vi "FID Main.vi"(8 "error in (no error)":errorcluster, 11 "User information":T1) -> (0 "error out":errorcluster)   [LabVIEW 2020]
uses:
  Controls/1775E_Authen_Level.ctl
  Controls/user_log.ctl
  <vilib>/Utility/miscctls.llb/LVPointTypeDef.ctl
  Controls/User_DB.ctl
  <vilib>/Instr/_visa.llb/VISA Configure Serial Port (Instr).vi
  <vilib>/addons/database/Connection.llb/Conn Execute.vi
  <vilib>/addons/database/Recordset.llb/Rec Fetch Recordset Data (R).vi
  <vilib>/addons/database/Recordset.llb/Rec Destroy - Connection.vi
  <vilib>/addons/database/NI_Database_API.lvlib
panel:
  in  "Hide":bool
  in  "Auth. Password":string caption="Password"
  in  "Change Password":bool
  out "State":string
  out "Device Info":string
  out "Numeric":i32
  in  "Re-enter Password":string
  in  "Password":string caption="New Password"
  in  "View Log":bool
  out "Cmd.":bool
  in  "Super User":bool
  in  "View All":bool
  out "String":string
  out "data":T1
  in  "Clock No.":string
  in  "Level":T2
  in  "User Name":string
  in  "ID Number":i16
  out "Finger Present?":bool
  out "Response":string
  in  "Delete All":bool
  in  "Delete":bool
  in  "Search":bool
  in  "Enroll":bool
  out "Status":string
  out "elements":u8[](array[numeric]) format="%.0x"
  in  "Stop":bool
  out "Buffer Out":string
  in  "write buffer":string="ï\u0001ÿÿÿÿ\u0001\u0000\u00034\u00008"
  out "Profile Image":picture
  in  "Image Location":path
  # "User Access Control"
  # "thumb finger"
  # "EF01 FFFF FFFF 0700 0700 0003 00A4 00B5"
  # "EF01 FFFF FFFF 0700 0709 0003 0028 0042"
  # "EF01 FFFF FFFF 0700 0700 0000 0065 0073"
  # "EF01 FFFF FFFF 0700 0700 0001 0084 0093"
  # "EF01 FFFF FFFF 0700 0709 0003 0002 001C"
  # "wrong finger"
  # "EF01 FFFF FFFF 0700 0703 0000 0000 0011"
  # "NO finger"
  # "EF01 FFFF FFFF 0700 0703 0000 0000 0011"
  # "EF01 FFFF FFFF 0700 0703 0000 0000 0011"
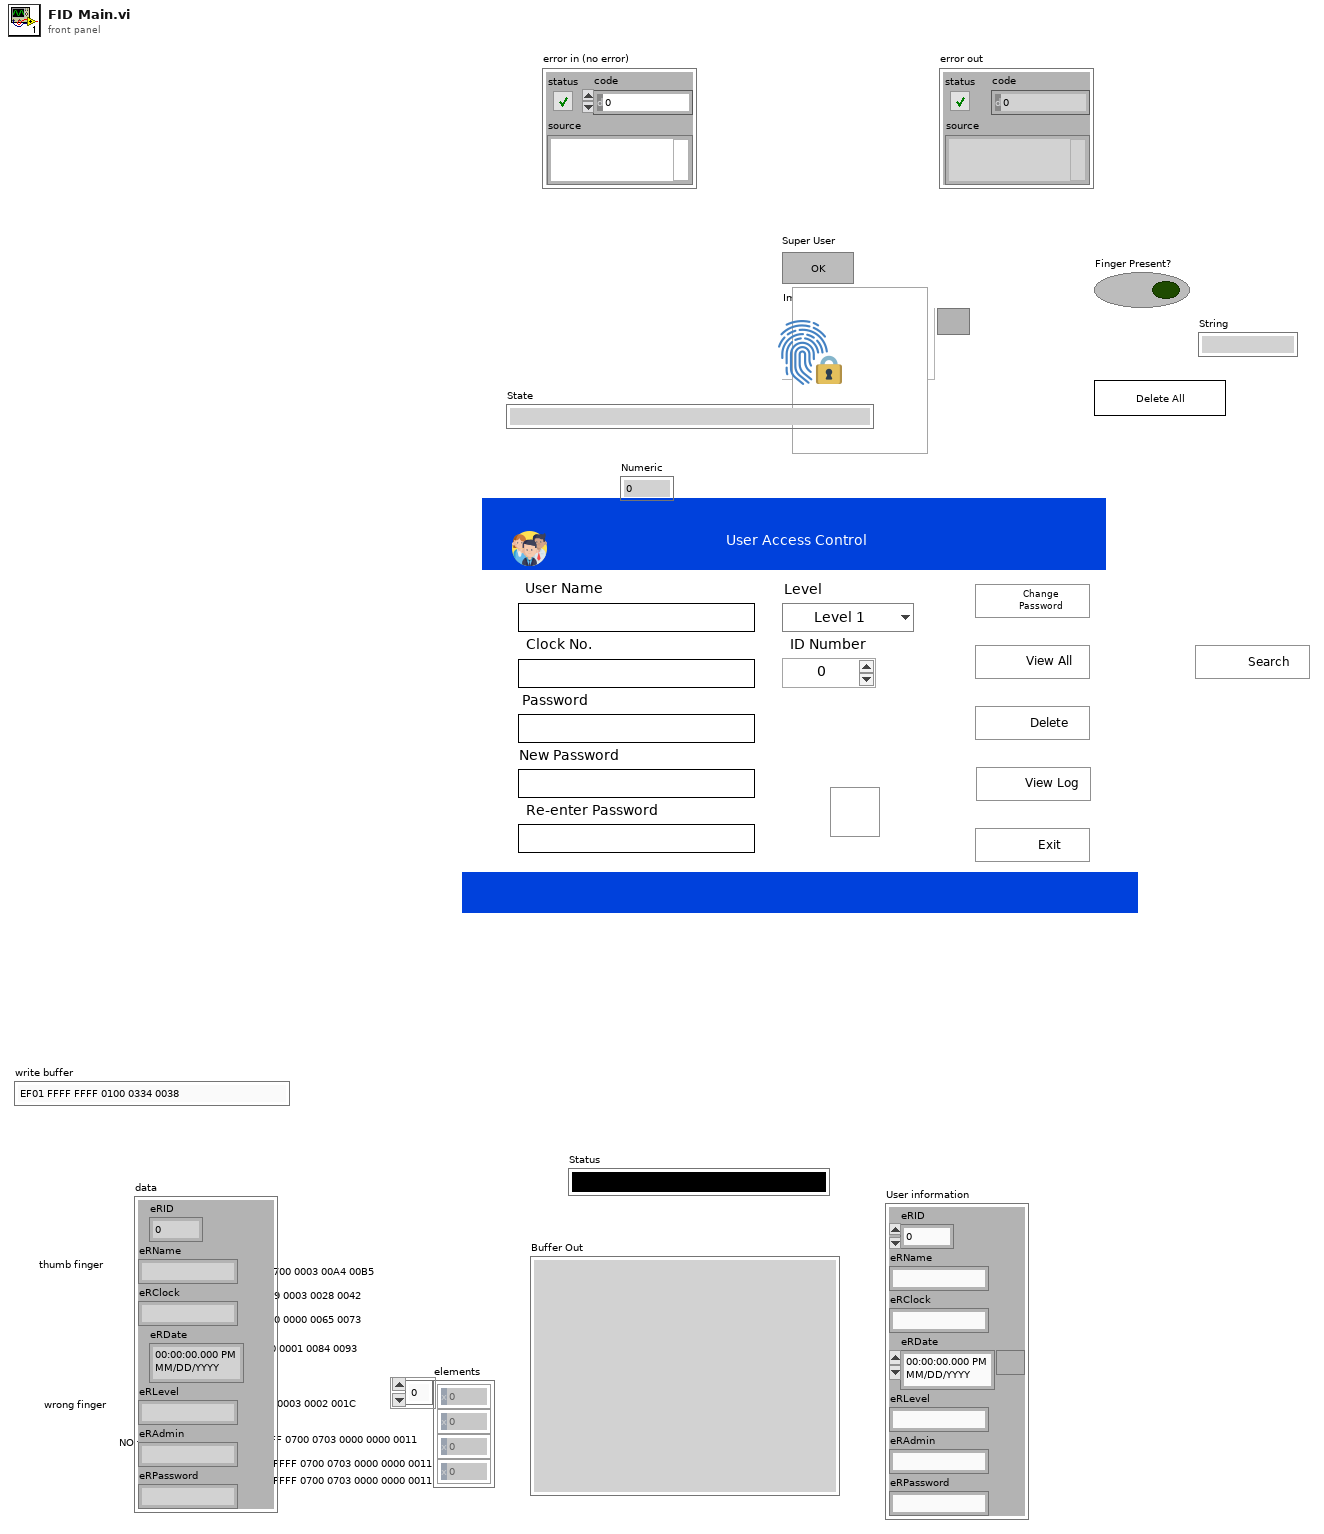
[diagram p1: front panel]
types:
  T1 = typedef "user_log.ctl" = cluster{"eRID":u16, "eRName":string, "eRClock":string, "eRDate":timestamp, "eRLevel":string, "eRAdmin":string, "eRPassword":string}
  T2 = typedef "1775E_Authen_Level.ctl" = enum16{"Level 1", "Level 2", "Level 3", "Level 4", "Super Level"}
  T3 = typedef "LVPointTypeDef.ctl" = cluster{"Horizontal":i16, "Vertical":i16}
  T4 = typedef "TD SQL.ctl" = cluster{"MS SQL Connection":T5, "UDL File":path, "Time":string, "DCODE":string, "WIP+1":i64, "MC No?":i32, "POKAYOKE?":bool, "Expected Result":string, "Result [Status]":string, "Clock":dbl, "RFID":string, "WIP Queue":refnum<queue>, "TS Parameter":T6, "Data_Queue":refnum<queue>[], "RFID Serial No.":string}
  T5 = typedef "NI_Database_API.lvlib/Conn ObjectReference.ctl" = refnum<k1>
  T6 = typedef "TS_Parameter.ctl" = cluster{"ProfitCenterCode":string, "LineCode":string, "WorkOrderNumber":string, "Model":string, "Model_with_Prefix":string, "VendorCode":string, "SetParameterDateCode":string, "PokaYoke":i32, "Target":i32, "Live_DateCode":string, "CustomerPartNumber":string, "Hand":string, "sBarcode":bool, "FCA":i32, "Ent_Stamp":timestamp, "STS_CD":dbl}
  T7 = typedef "User_DB.ctl" = cluster{"eRID":u16, "eRName":string, "eRClock":string, "eRDate":timestamp, "eRLevel":string, "eRAdmin":string, "eRPassword":string, "eRPurpose":string}
  T8 = typedef "NI_Database_API.lvlib/Rec ObjectReference.ctl" = refnum<k1>
  T9 = typedef "imagedata.ctl" = cluster{"image type":i32, "image depth":i32, "image":u8[], "mask":u8[], "colors":u32[], "Rectangle":cluster{"left":i16, "top":i16, "right":i16, "bottom":i16}}
  T10 = typedef "LVBoundsTypeDef.ctl" = cluster{"Width":u32, "Height":u32}
  T11 = cluster{"left":i16, "top":i16, "right":i16, "bottom":i16}
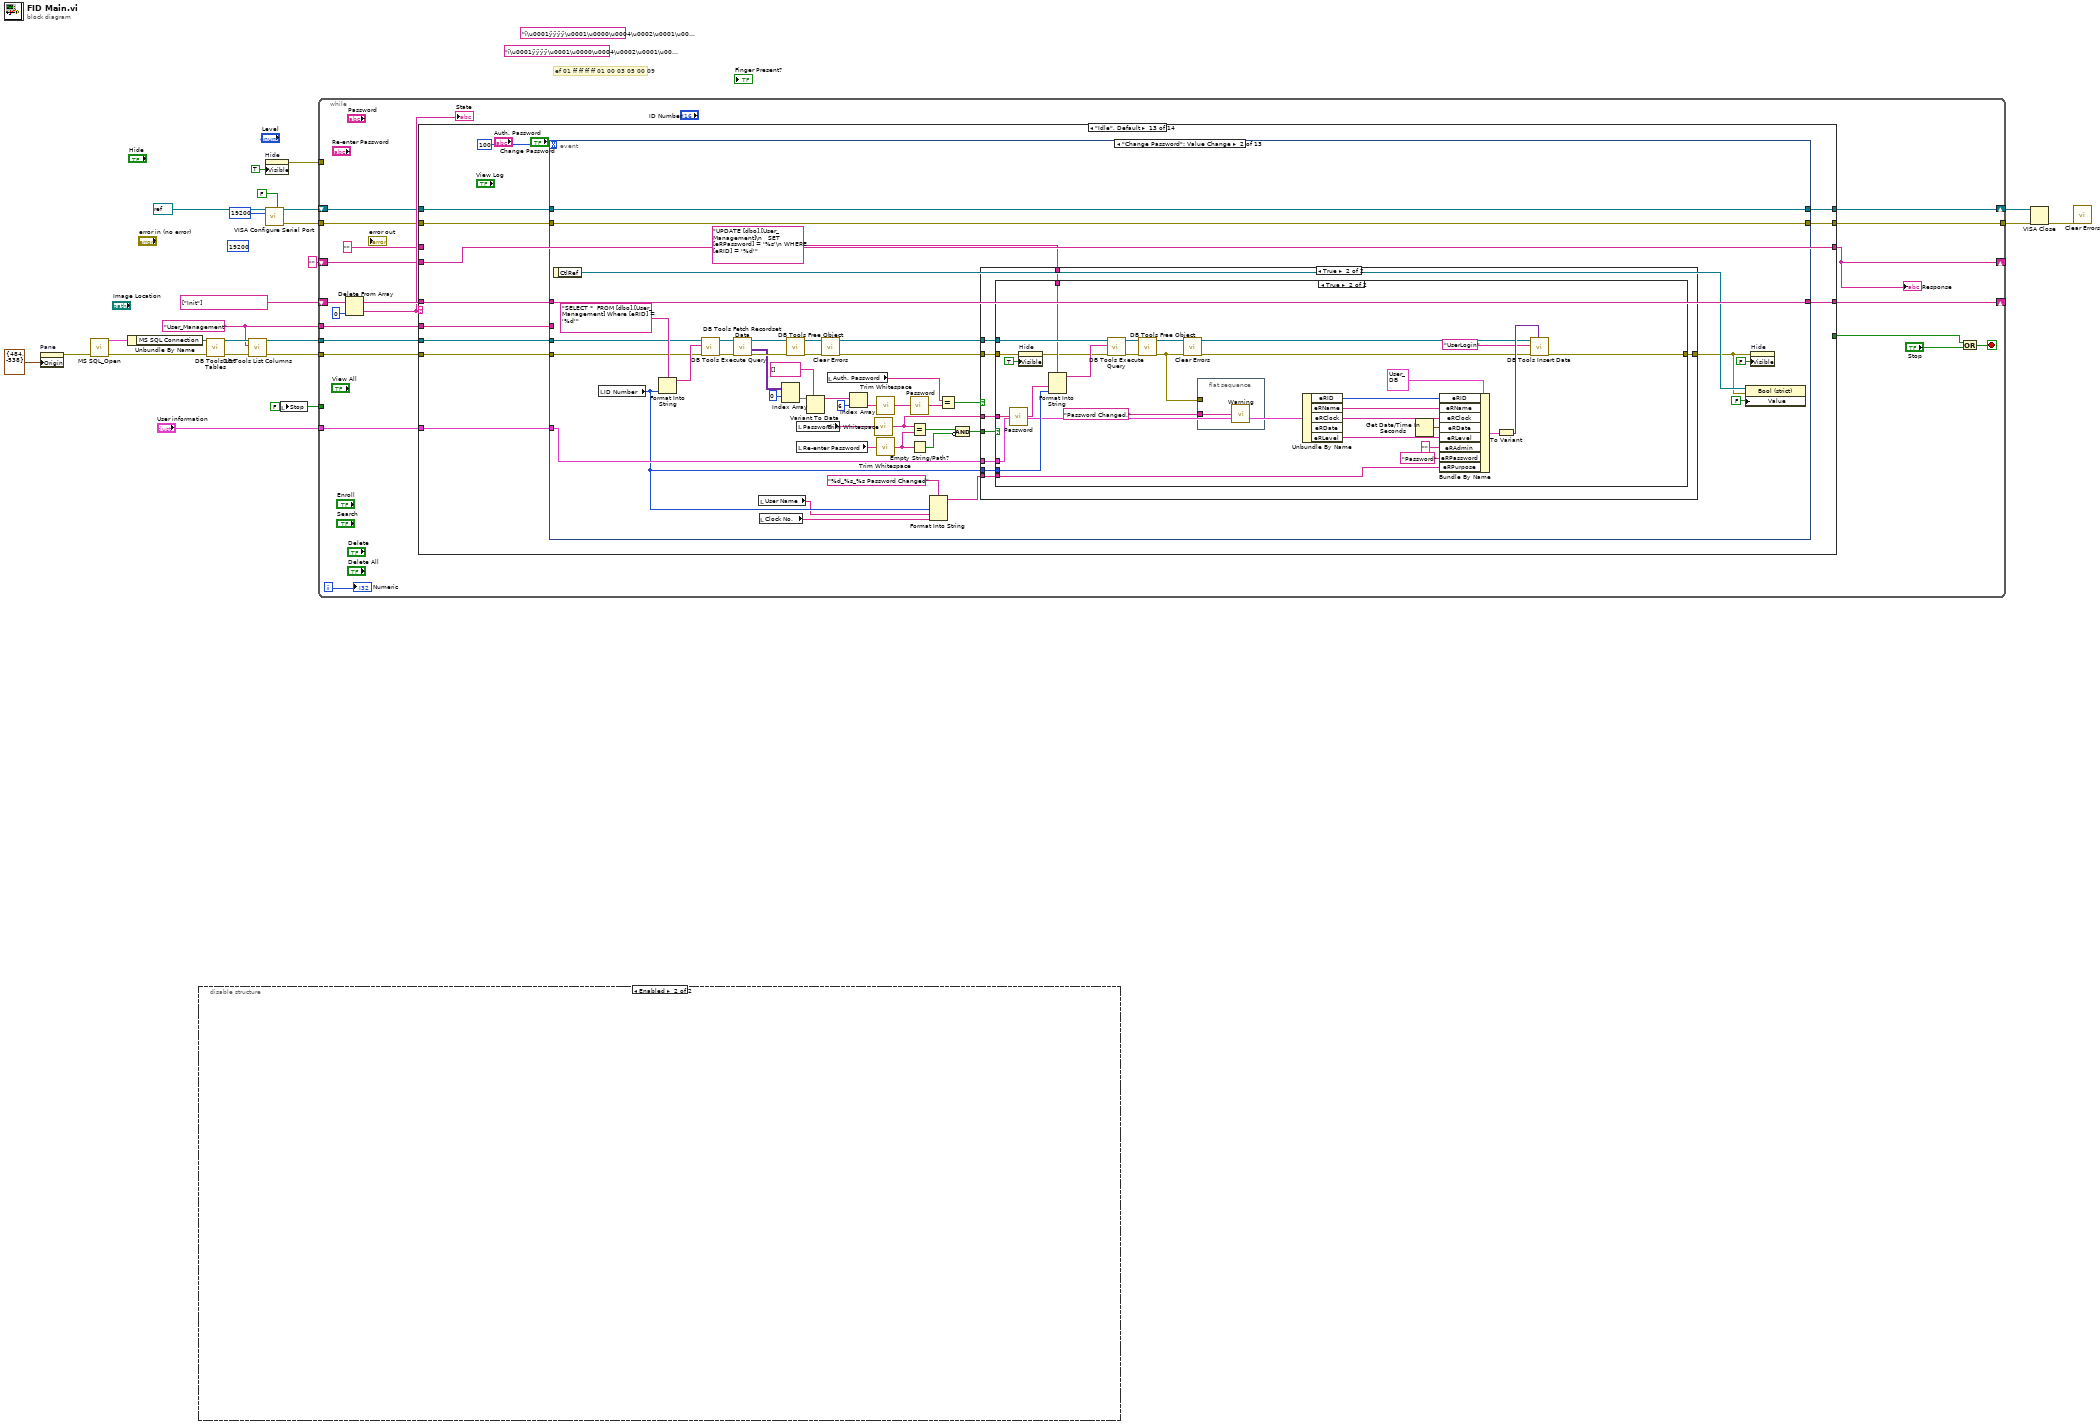
[diagram p0: block diagram]
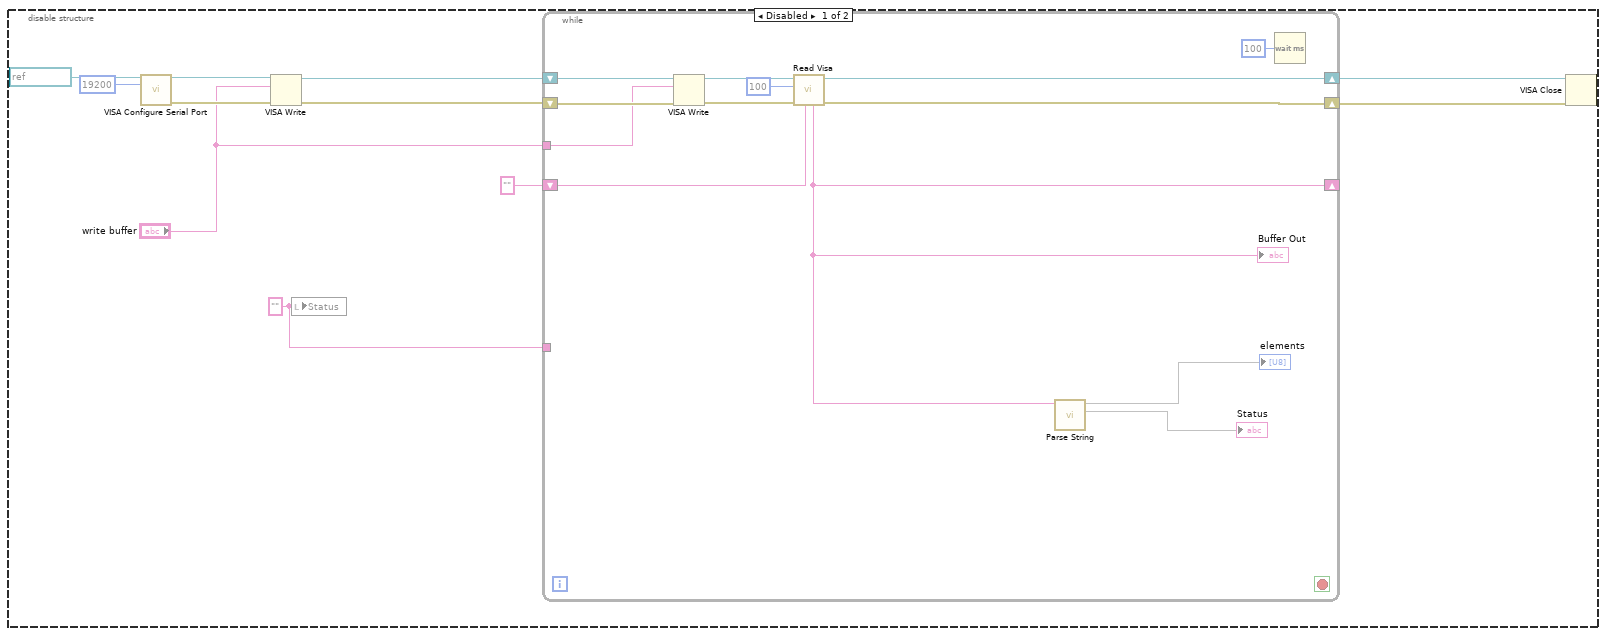
[diagram p2: hidden frame]
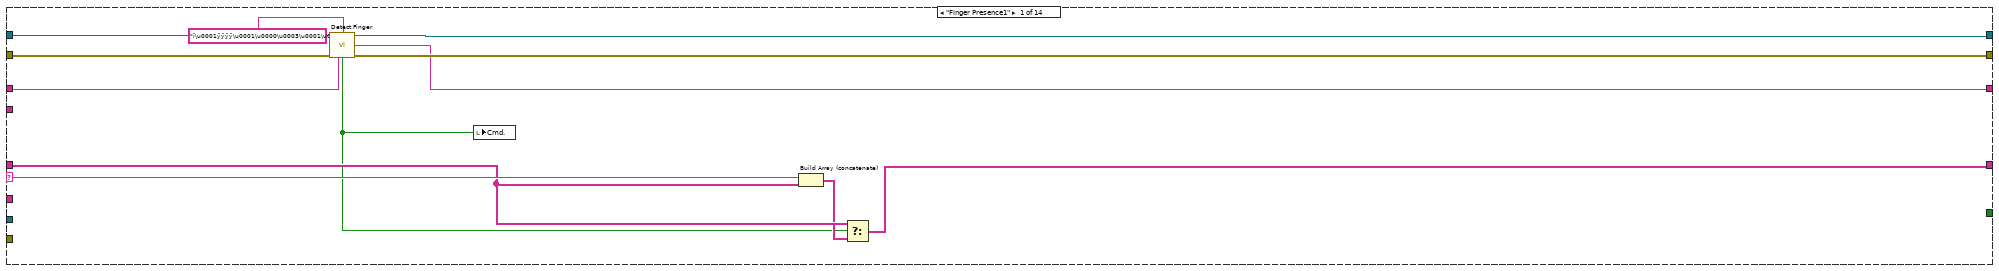
[diagram p3: hidden frame]
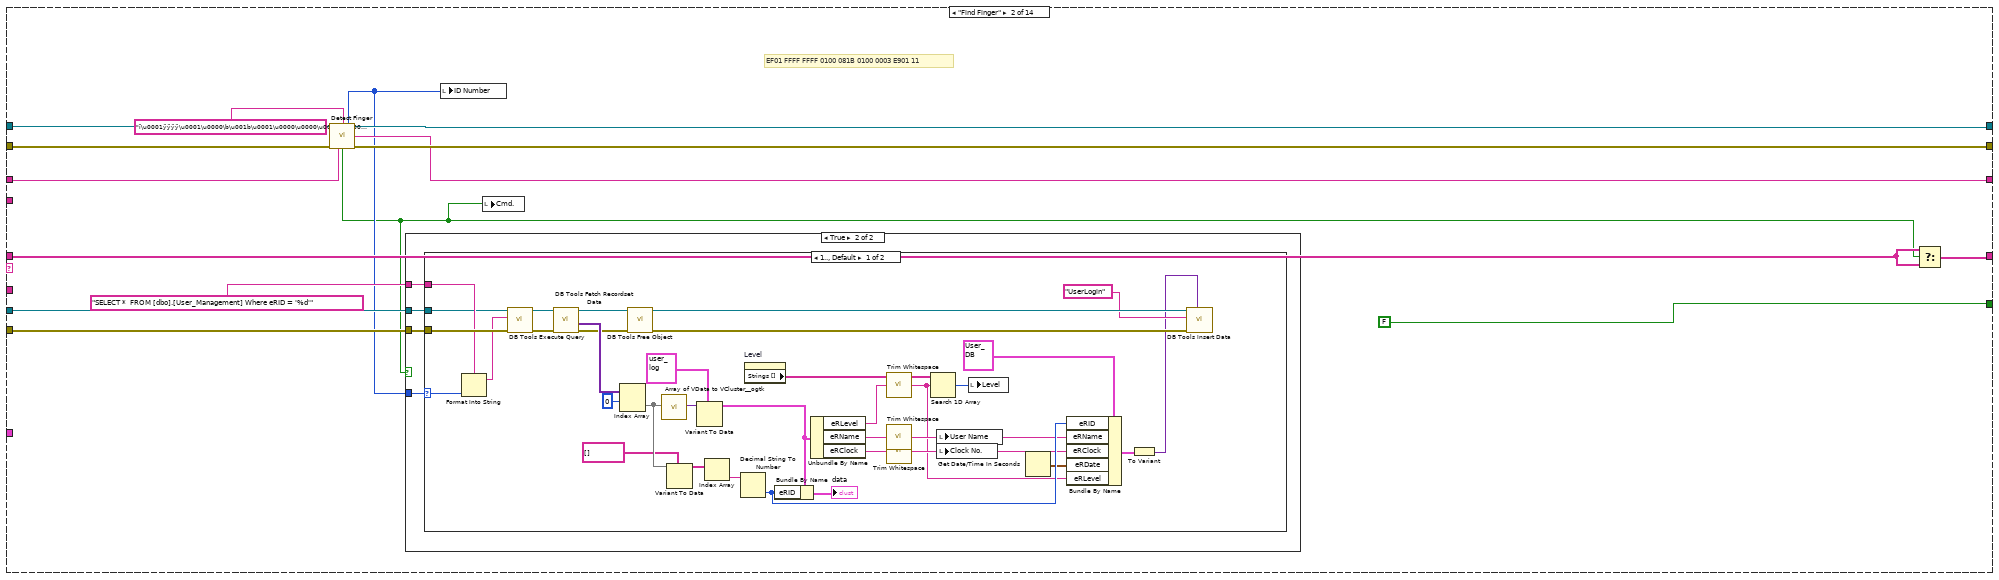
[diagram p4: hidden frame]
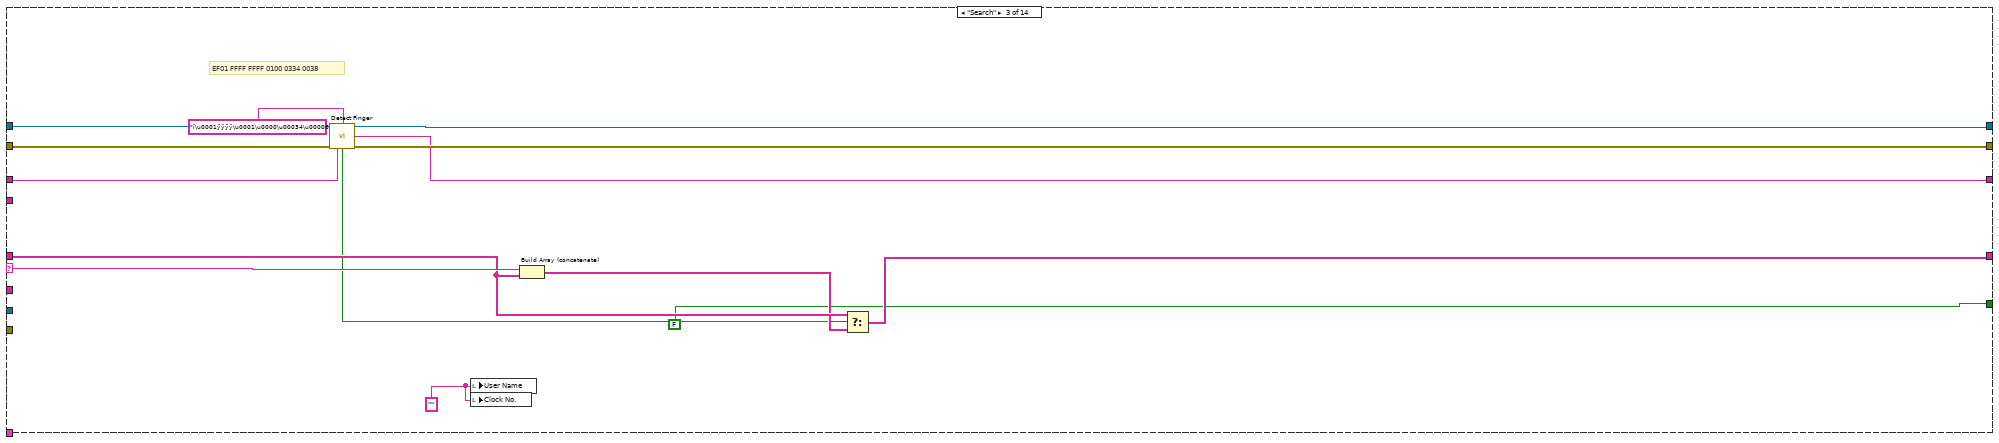
[diagram p7: hidden frame]
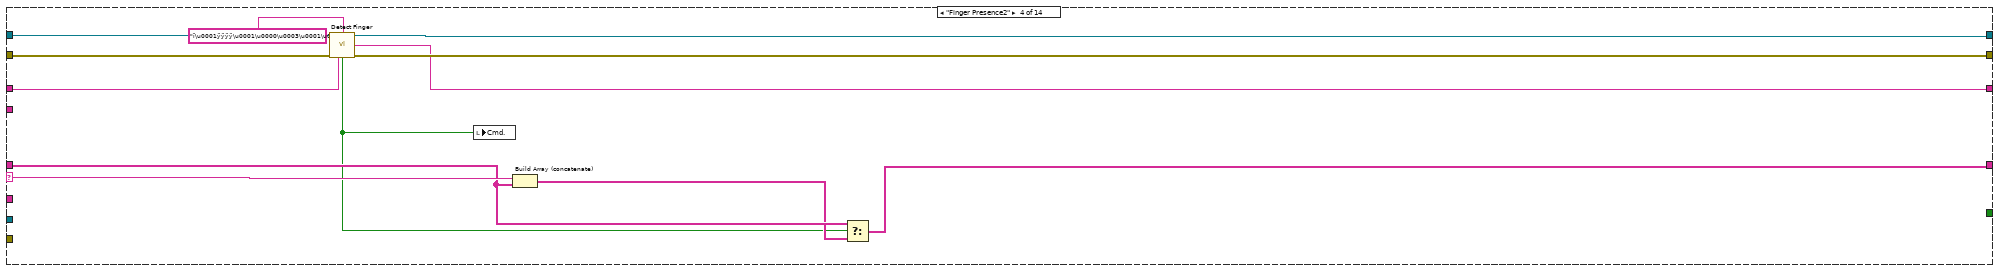
[diagram p8: hidden frame]
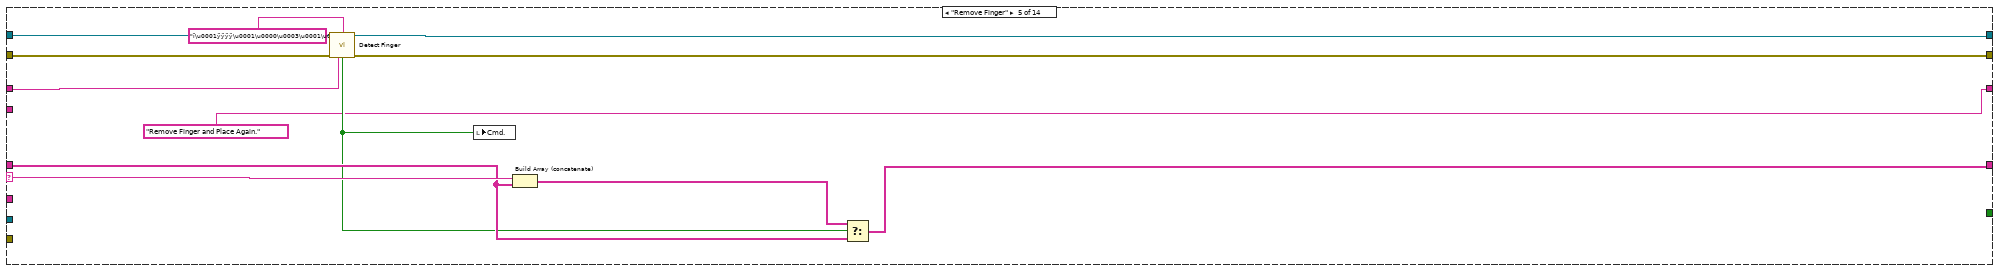
[diagram p9: hidden frame]
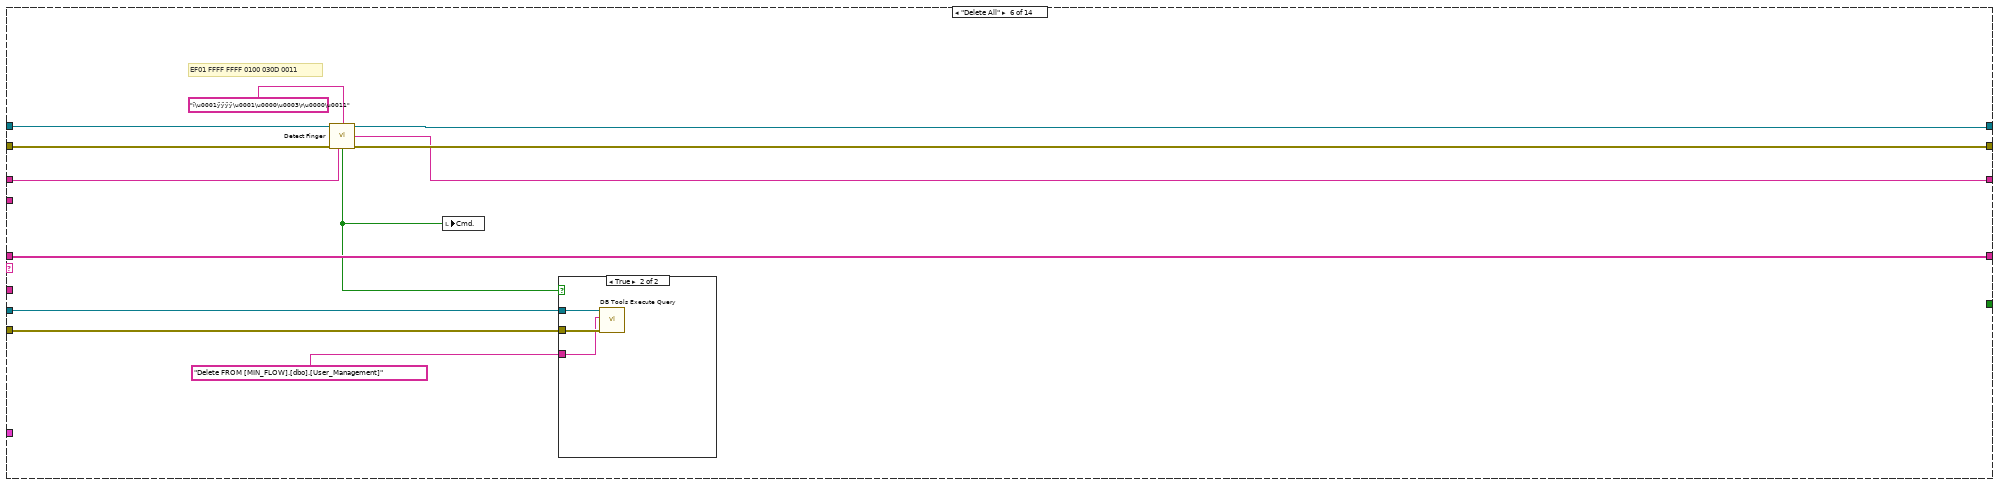
[diagram p10: hidden frame]
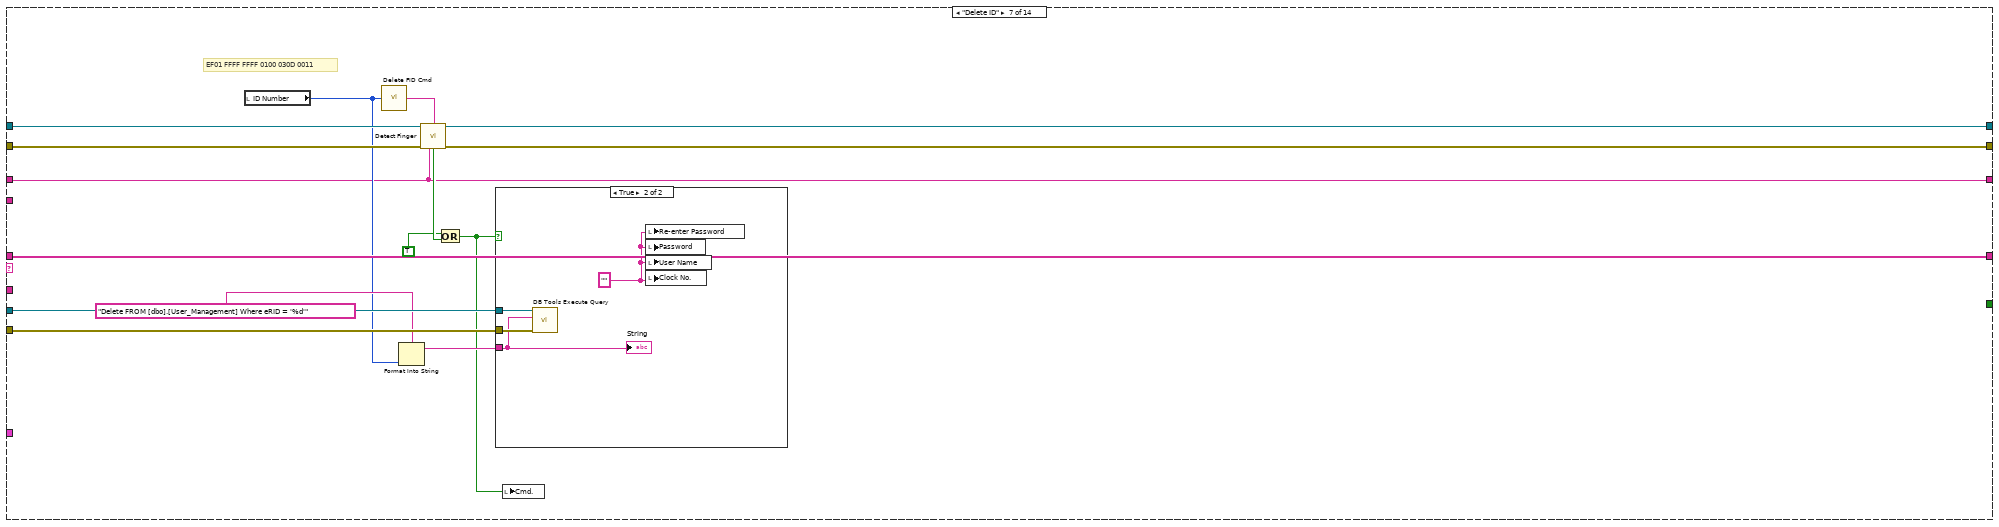
[diagram p12: hidden frame]
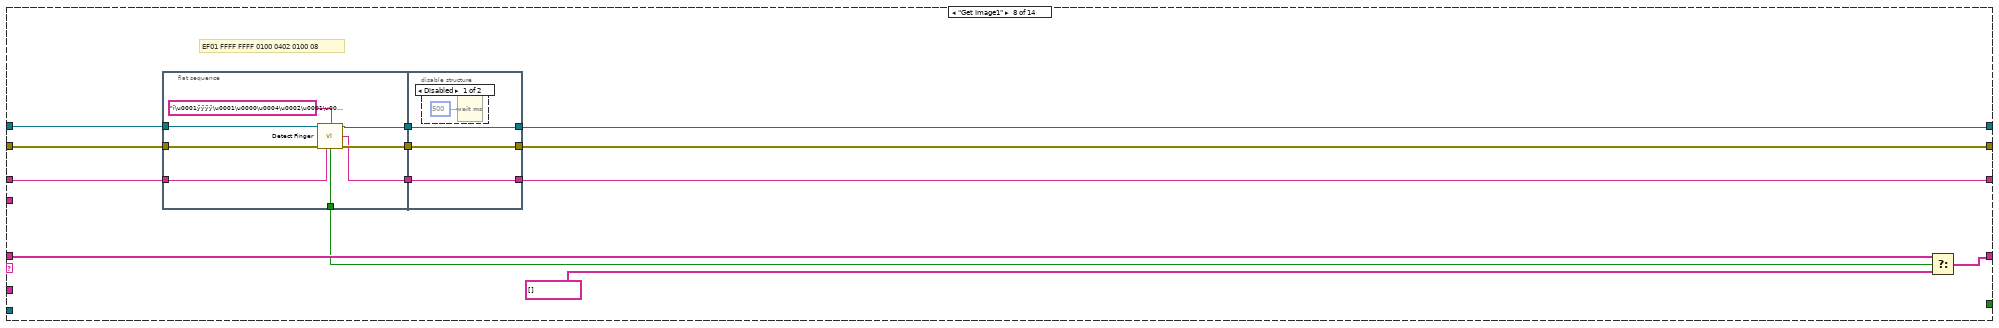
[diagram p14: hidden frame]
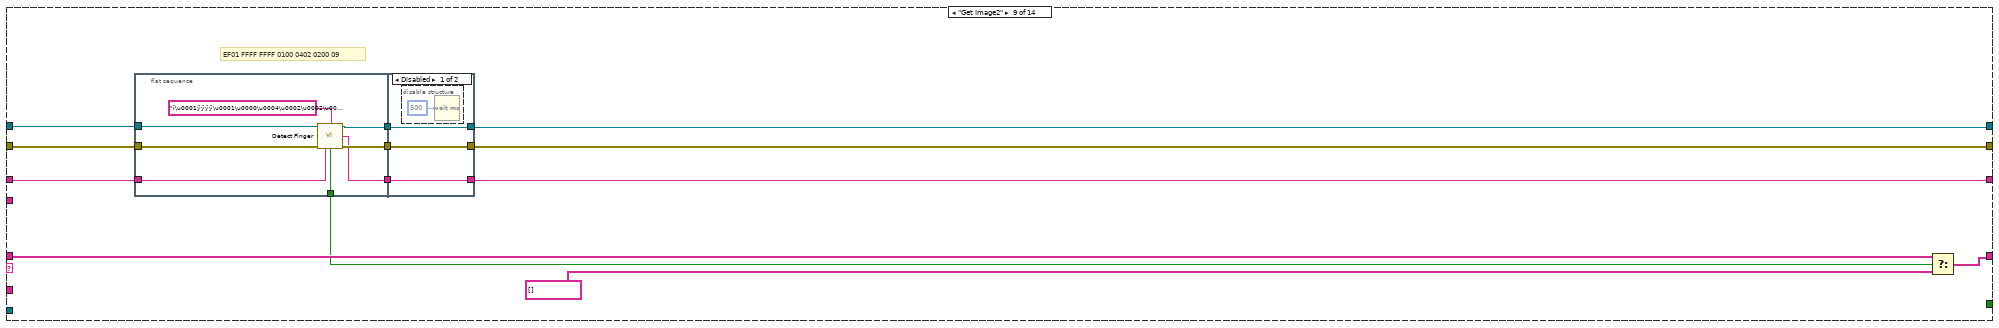
[diagram p16: hidden frame]
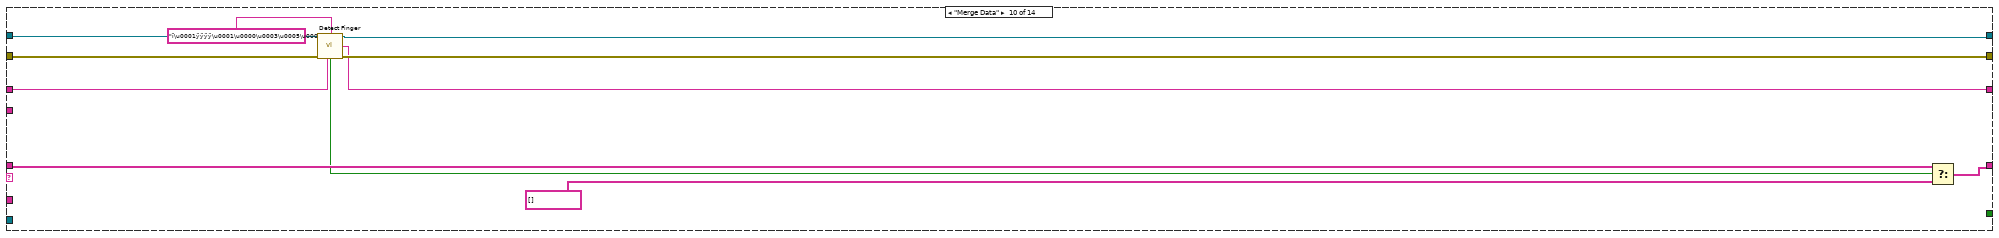
[diagram p18: hidden frame]
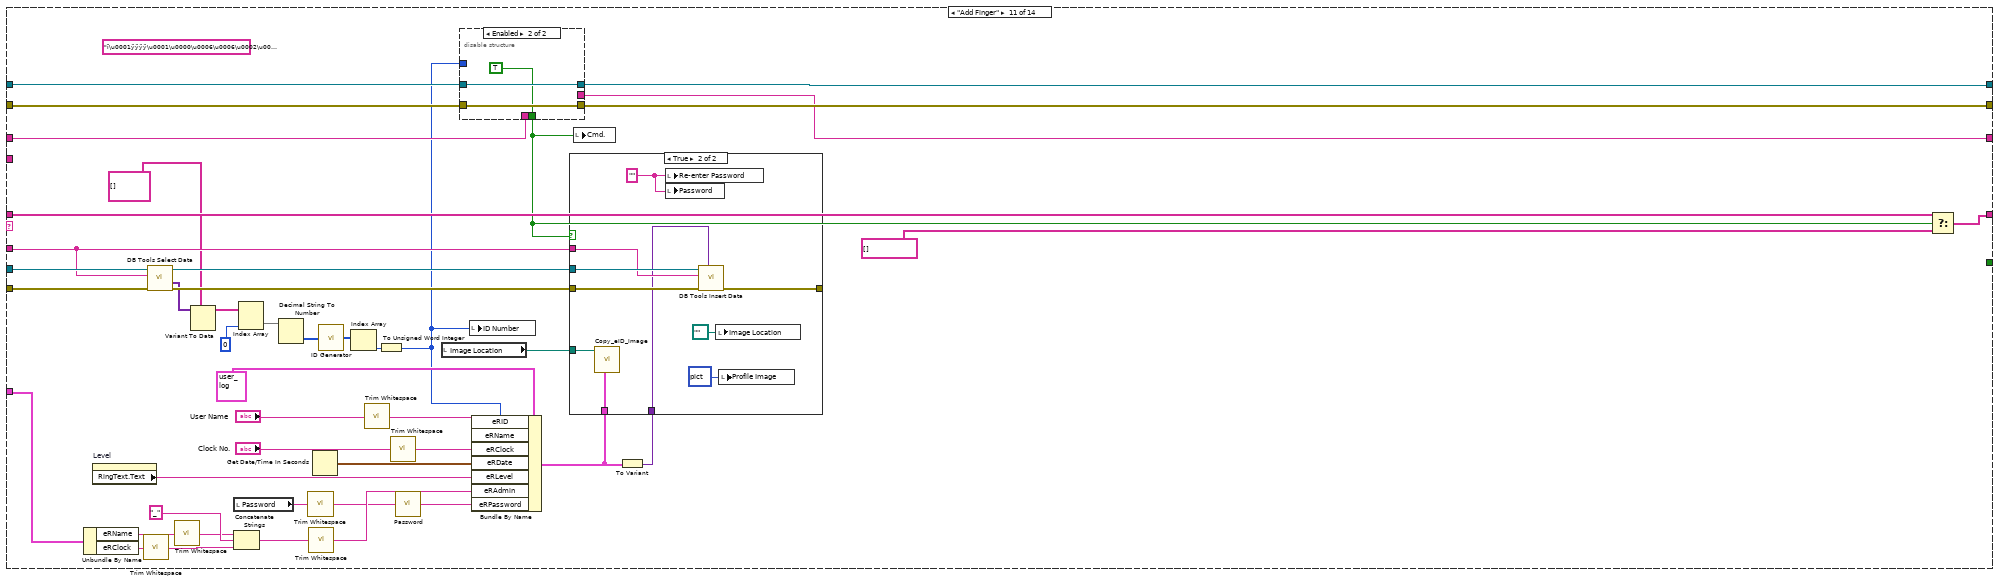
[diagram p19: hidden frame]
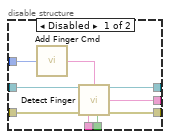
[diagram p20: hidden frame]
diagram:
  (unwired) u32 19200 ("baud rate (9600)")
  w11 = FALSE ("Stop")
  w12 = "User_Management" ("table")
  (unwired) "ï\u0001ÿÿÿÿ\u0001\u0000\u0004\u0002\u0001\u0000\b" ("write buffer")
  (unwired) "ï\u0001ÿÿÿÿ\u0001\u0000\u0004\u0002\u0001\u0000\b" ("write buffer")
  # "ef 01 ff ff ff ff 01 00 03 05 00 09"
  n1 = property on="Pane" class="Pane"("Origin"=T3 {"Horizontal"=484, "Vertical"=-538}) -> (error out=w2:errorcluster)  [unwired: 2 in, 1 out]
  n2 = call "MS SQL_Open.vi"("error in (no error)"=w2) -> ("error out"=w1:errorcluster, "Ref Out"=w4:T4)  [unwired: 8 in, 1 out]
  n3 = Unbundle By Name(w4) -> ("MS SQL Connection"=w3:T5)
  n4 = disable-structure shown="Enabled" {
    frame Disabled {
      w25 = "" ("Status")
      n5 = call-poly "VISA Configure Serial Port"("VISA resource name"=refnum<visa-resource-name> "COM6", "baud rate (9600)"=u32 19200) -> ("VISA resource name out"=w31:refnum<visa-resource-name>, "error out"=w29:errorcluster)  [unwired: 12 in]
      n6 = VISA Write(VISA resource name=w31, write buffer="write buffer", error in (no error)=w29) -> (VISA resource name out=w30:refnum<visa-resource-name>, error out=w28:errorcluster)  [unwired: 1 out]
      n7 = local write "Status"(w25) -> ()
      n8 = while {
        shift-right: [w49] -> w33
        shift-left: w30 -> [w43]
        shift-right: [w48] -> w32
        shift-left: w28 -> [w42]
        shift-right: [w38] -> _
        shift-left: "" ("Buffer Out") -> [w44]
        tunnel: "write buffer" -> [w39]
        tunnel: w25 -> [_]
        stop <- w46 stop-if-true
        n9 = VISA Write(VISA resource name=w43, write buffer=w39, error in (no error)=w42) -> (VISA resource name out=w40:refnum<visa-resource-name>, error out=w41:errorcluster)  [unwired: 1 out]
        n10 = call <userlib>:"Read Visa.vi"("Buffer In"=w44, "error in (no error)"=w41, "delay before read (ms)"=u32 100, "VISA Refnum in"=w40) -> ("error out"=w48:errorcluster, "VISA Refnum out"=w49:refnum<visa-resource-name>, "Buffer Out"=w38:string)  [unwired: 5 in]
        "Buffer Out" <- w38
        n11 = call "Parse String.vi"("Ack package"=w38) -> (2:→"Status", 3:→"elements")  [unwired: 7 in, 2 out]
        n12 = Wait (ms)(milliseconds to wait=u32 100) -> ()  [unwired: 1 out]
      }
      n13 = VISA Close(VISA resource name=w33, error in (no error)=w32) -> ()  [unwired: 1 out]
    }
    frame Enabled {
    }
  }
  n14 = call <vilib>:"DB Tools List Tables.vi"("error in (no error)"=w1, "connection reference"=w3) -> ("error out"=w15:errorcluster, "connection reference out"=w16:T5)  [unwired: 3 in, 1 out]
  n15 = call <vilib>:"DB Tools List Columns.vi"("error in (no error)"=w15, "table"=w12, "connection reference"=w16) -> ("error out"=w13:errorcluster, "connection reference out"=w14:T5)  [unwired: 1 in, 2 out]
  n16 = property on="Hide" class="Bool"("Visible"=TRUE) -> (error out=w7:errorcluster)  [unwired: 2 in, 1 out]
  n17 = call-poly "VISA Configure Serial Port"("VISA resource name"=refnum<visa-resource-name> refnum, "Enable Termination\nChar (T)"=FALSE ("Enable Termination\nChar (T)"), "baud rate (9600)"=u32 19200) -> ("VISA resource name out"=w22:refnum<visa-resource-name>, "error out"=w21:errorcluster)  [unwired: 11 in]
  n18 = local write "Stop"(w11) -> ()
  n19 = while {
    shift-right: [w68] -> _
    shift-left: string[] ["Init"] -> [w69]
    tunnel: w21 -> [w51]
    shift-right: [w67] -> w19
    shift-left: w22 -> [w50]
    shift-right: [w57] -> _
    shift-left: "" ("Buffer Out") -> [w58]
    tunnel: [w64] -> w18
    tunnel: w14 -> [w56]
    tunnel: w13 -> [w55]
    tunnel: w12 -> [w54]
    tunnel: w11 -> [_]
    tunnel: "User information" -> [w53]
    tunnel: w7 -> [_]
    i -> [w52]
    stop <- w62 stop-if-true
    n20 = Delete From Array(array=w69, index=0) -> (deleted portion=w61:string, array with subset deleted=w65:string[])  [unwired: 1 in]
    "State" <- w61
    n21 = case shown="\"Idle\", Default" w61 {
      selector: w61 -> [w81 _ w149 w161 w173 _ _ _ _ _ _ _ _ _]
      tunnel: w65 -> [w80 w87 w148 w160 w172 w178 w198 w220 w245 w268 w313 w336 w350 w590]
      tunnel: [w78 w96 w146 w158 w170 w178 w198 w219 w244 w267 w312 w336 w349 w590] -> w68
      tunnel: w50 -> [w77 w95 w145 w157 w169 w185 w203 w217 w242 w265 w310 w339 w348 w588]
      tunnel: w51 -> [w76 w94 w144 w156 w168 w184 w202 w216 w241 w264 w309 w338 w347 w585]
      tunnel: [w74 w92 w142 w154 w166 w182 w200 w215 w240 w263 w308 w339 w346 w587] -> w67
      tunnel: [w75 w93 w143 w155 w167 w183 w201 w214 w239 w262 w307 w338 w345 w584] -> w64
      tunnel: [w73 w91 w141 w153 "Remove Finger and Place Again." ("Response") w181 w189 w212 w237 w260 w306 w337 w344 w589] -> w57
      tunnel: "" ("Buffer Out") -> [w70 w89 w137 w150 w163 w179 w189 w208 w233 w258 w305 w337 _ w586]
      tunnel: [_ FALSE ("Stop") FALSE ("Stop") _ _ _ _ _ _ _ _ _ _ _] -> w60
      tunnel: w58 -> [_ _ _ _ _ _ _ _ _ _ _ _ w344 _]
      tunnel: w56 -> [_ w86 _ _ _ w177 w197 _ _ _ w304 _ w343 _]
      tunnel: w55 -> [_ w85 _ _ _ w176 w196 _ _ _ w303 _ w342 _]
      tunnel: w54 -> [_ _ _ _ _ _ _ _ _ _ w299 _ w341 _]
      tunnel: w53 -> [_ _ _ _ _ _ _ _ _ _ w282 _ w340 _]
      frame "Finger Presence1" {
        n22 = call "Detect Finger.vi"("VISA Refnum in"=w77, "Cmd"="ï\u0001ÿÿÿÿ\u0001\u0000\u0003\u0001\u0000\u0005" ("write buffer"), "error in (no error)"=w76, "Buffer In"=w70) -> ("VISA Refnum out"=w74:refnum<visa-resource-name>, "Response"=w73:string, "Cmd Suceed?"=w71:bool, "error out"=w75:errorcluster)  [unwired: 6 in, 2 out]
        n23 = local write "Cmd."(w71) -> ()
        n24 = Build Array (concatenate)(w81, w80) -> (w79:string[])
        n25 = Select(t=w80, s=w71, f=w79) -> (s? t:f=w78:string[])
      }
      frame "Find Finger" {
        # "EF01 FFFF FFFF 0100 081B 0100 0003 E901 11"
        n26 = call "Detect Finger.vi"("VISA Refnum in"=w95, "Cmd"="ï\u0001ÿÿÿÿ\u0001\u0000\b\u001b\u0001\u0000\u0000\u0003é\u0001\u0011" ("write buffer"), "error in (no error)"=w94, "Buffer In"=w89) -> ("ID"=w83:i16, "VISA Refnum out"=w92:refnum<visa-resource-name>, "Response"=w91:string, "Cmd Suceed?"=w82:bool, "error out"=w93:errorcluster)  [unwired: 6 in, 1 out]
        n27 = case shown="True" w82 {
          tunnel: w86 -> [_ w100]
          tunnel: w85 -> [_ w99]
          tunnel: "SELECT *  FROM [dbo].[User_Management] Where eRID = '%d'" ("SQL query") -> [_ w98]
          tunnel: w83 -> [_ w97]
          frame False {
          }
          frame True {
            n28 = case shown="1.., Default" w97 {
              selector: w97 -> [w132 _]
              tunnel: w100 -> [w114 _]
              tunnel: w99 -> [w134 _]
              tunnel: w98 -> [w133 _]
              frame 1.., Default {
                n29 = Format Into String(format string=w133, w132) -> (resulting string=w131:string)  [unwired: 2 in, 1 out]
                n30 = call-poly <vilib>:"DB Tools Execute Query.vi"("error in (no error)"=w134, "SQL query"=w131, "connection reference"=w114) -> ("error out"=w135:errorcluster, "recordset reference"=w115:T8)  [unwired: 5 in]
                n31 = call-poly <vilib>:"DB Tools Fetch Recordset Data.vi"("error in (no error)"=w135, "recordset reference"=w115) -> ("error out"=w111:errorcluster, "recordset data"=w127:variant[][], "recordset reference out"=w113:T8)  [unwired: 3 in]
                n32 = Index Array(array=w127, index (row)=0 ("disabled index (col)")) -> (element=w126:variant[])  [unwired: 1 in]
                n33 = call-poly <vilib>:"DB Tools Free Object.vi"("error in (no error)"=w111, "recordset reference"=w113) -> ("error out"=w110:errorcluster, "connection reference"=w112:T5)  [unwired: 8 in]
                n34 = call <userlib>:"Array of VData to VCluster__ogtk.vi"("Array"=w126) -> ("VCluster"=w129:variant)  [unwired: 9 in, 1 out]
                n35 = Variant To Data(type=string[] [], Variant=w126) -> (data=w124:string[])  [unwired: 1 in, 1 out]
                n36 = Variant To Data(type=T1 {"eRID"=0, "eRName"="", "eRClock"="", "eRDate"=timestamp(0 s since 1904-01-01), "eRLevel"="", "eRAdmin"="", "eRPassword"=""} ("Cluster"), Variant=w129) -> (data=w121:T1)  [unwired: 1 in, 1 out]
                n37 = Index Array(array=w124) -> (element=w123:string)  [unwired: 1 in]
                n38 = Decimal String To Number(string=w123) -> (number=w107:i32)  [unwired: 2 in, 1 out]
                n39 = property on="Level" class="Enum (strict)"() -> ("Strings []"=w116:string[])  [unwired: 2 in, 2 out]
                n40 = Bundle By Name(cluster=w121, "eRID"=w107) -> (→"data":T1)
                n41 = Unbundle By Name(w121) -> ("eRLevel"=w120:string, "eRName"=w118:string, "eRClock"=w117:string)
                n42 = call <vilib>:"Trim Whitespace.vi"("string"=w120) -> ("trimmed string"=w104:string)  [unwired: 1 in]
                n43 = call <vilib>:"Trim Whitespace.vi"("string"=w118) -> ("trimmed string"=w106:string)  [unwired: 1 in]
                n44 = call <vilib>:"Trim Whitespace.vi"("string"=w117) -> ("trimmed string"=w105:string)  [unwired: 1 in]
                n45 = Search 1D Array(1D array=w116, element=w104) -> (index of element=w119:i32)  [unwired: 1 in]
                n46 = local write "User Name"(w106) -> ()
                n47 = local write "Clock No."(w105) -> ()
                n48 = local write "Level"(w119) -> ()
                n49 = Get Date/Time In Seconds() -> (seconds since 1Jan1904=w103:timestamp)
                n50 = Bundle By Name(cluster=T7 {"eRID"=0, "eRName"="", "eRClock"="", "eRDate"=timestamp(0 s since 1904-01-01), "eRLevel"="", "eRAdmin"="", "eRPassword"="", "eRPurpose"=""} ("Cluster"), "eRID"=w107, "eRName"=w106, "eRClock"=w105, "eRDate"=w103, "eRLevel"=w104) -> (w102:T7)
                n51 = To Variant(anything=w102) -> (Variant=w101:variant)
                n52 = call <vilib>:"DB Tools Insert Data.vi"("data"=w101, "error in (no error)"=w110, "table"="UserLogin", "connection reference"=w112) -> ()  [unwired: 6 in, 2 out]
              }
              frame -1, 0 {
              }
            }
          }
        }
        n53 = local write "ID Number"(w83) -> ()
        n54 = local write "Cmd."(w82) -> ()
        n55 = Select(t=w87, s=w82, f=w87) -> (s? t:f=w96:string[])
      }
      frame "Search" {
        w136 = "" ("User Name")
        # "EF01 FFFF FFFF 0100 0334 0038"
        n56 = call "Detect Finger.vi"("VISA Refnum in"=w145, "Cmd"="ï\u0001ÿÿÿÿ\u0001\u0000\u00034\u00008" ("write buffer"), "error in (no error)"=w144, "Buffer In"=w137) -> ("VISA Refnum out"=w142:refnum<visa-resource-name>, "Response"=w141:string, "Cmd Suceed?"=w139:bool, "error out"=w143:errorcluster)  [unwired: 6 in, 2 out]
        n57 = local write "User Name"(w136) -> ()
        n58 = local write "Clock No."(w136) -> ()
        n59 = Build Array (concatenate)(w149, w148) -> (w147:string[])
        n60 = Select(t=w148, s=w139, f=w147) -> (s? t:f=w146:string[])
      }
      frame "Finger Presence2" {
        n61 = call "Detect Finger.vi"("VISA Refnum in"=w157, "Cmd"="ï\u0001ÿÿÿÿ\u0001\u0000\u0003\u0001\u0000\u0005" ("write buffer"), "error in (no error)"=w156, "Buffer In"=w150) -> ("VISA Refnum out"=w154:refnum<visa-resource-name>, "Response"=w153:string, "Cmd Suceed?"=w151:bool, "error out"=w155:errorcluster)  [unwired: 6 in, 2 out]
        n62 = local write "Cmd."(w151) -> ()
        n63 = Build Array (concatenate)(w161, w160) -> (w159:string[])
        n64 = Select(t=w160, s=w151, f=w159) -> (s? t:f=w158:string[])
      }
      frame "Remove Finger" {
        n65 = call "Detect Finger.vi"("VISA Refnum in"=w169, "Cmd"="ï\u0001ÿÿÿÿ\u0001\u0000\u0003\u0001\u0000\u0005" ("write buffer"), "error in (no error)"=w168, "Buffer In"=w163) -> ("VISA Refnum out"=w166:refnum<visa-resource-name>, "Cmd Suceed?"=w164:bool, "error out"=w167:errorcluster)  [unwired: 6 in, 3 out]
        n66 = local write "Cmd."(w164) -> ()
        n67 = Build Array (concatenate)(w173, w172) -> (w171:string[])
        n68 = Select(t=w171, s=w164, f=w172) -> (s? t:f=w170:string[])
      }
      frame "Delete All" {
        # "EF01 FFFF FFFF 0100 030D 0011"
        n69 = call "Detect Finger.vi"("VISA Refnum in"=w185, "Cmd"="ï\u0001ÿÿÿÿ\u0001\u0000\u0003\r\u0000\u0011" ("write buffer"), "error in (no error)"=w184, "Buffer In"=w179) -> ("VISA Refnum out"=w182:refnum<visa-resource-name>, "Response"=w181:string, "Cmd Suceed?"=w174:bool, "error out"=w183:errorcluster)  [unwired: 6 in, 2 out]
        n70 = local write "Cmd."(w174) -> ()
        n71 = case shown="True" w174 {
          tunnel: w177 -> [_ w188]
          tunnel: w176 -> [_ w187]
          tunnel: "Delete FROM [MIN_FLOW].[dbo].[User_Management]" ("SQL query") -> [_ w186]
          frame False {
          }
          frame True {
            n72 = call-poly <vilib>:"DB Tools Execute Query.vi"("error in (no error)"=w187, "SQL query"=w186, "connection reference"=w188) -> ()  [unwired: 5 in, 2 out]
          }
        }
      }
      frame "Delete ID" {
        # "EF01 FFFF FFFF 0100 030D 0011"
        n73 = local read "ID Number"() -> (w193:i16)
        n74 = call "Delete FID Cmd.vi"("ID"=w193) -> ("Cmd"=w199:string)
        n75 = Format Into String(format string="Delete FROM [dbo].[User_Management] Where eRID = '%d'" ("SQL query"), w193) -> (resulting string=w194:string)  [unwired: 2 in, 1 out]
        n76 = call "Detect Finger.vi"("VISA Refnum in"=w203, "Cmd"=w199, "error in (no error)"=w202, "Buffer In"=w189) -> ("VISA Refnum out"=w200:refnum<visa-resource-name>, "Cmd Suceed?"=w192:bool, "error out"=w201:errorcluster)  [unwired: 6 in, 3 out]
        n77 = Compound Arithmetic op=OR(TRUE ("value"), w192) -> (w191:bool)
        n78 = case shown="True" w191 {
          tunnel: w197 -> [_ w207]
          tunnel: w196 -> [_ w206]
          tunnel: w194 -> [_ w205]
          frame False {
          }
          frame True {
            w204 = "" ("User Name")
            n79 = call-poly <vilib>:"DB Tools Execute Query.vi"("error in (no error)"=w206, "SQL query"=w205, "connection reference"=w207) -> ()  [unwired: 5 in, 2 out]
            n80 = local write "Re-enter Password"(w204) -> ()
            n81 = local write "Password"(w204) -> ()
            n82 = local write "User Name"(w204) -> ()
            n83 = local write "Clock No."(w204) -> ()
            "String" <- w205
          }
        }
        n84 = local write "Cmd."(w191) -> ()
      }
      frame "Get Image1" {
        # "EF01 FFFF FFFF 0100 0402 0100 08"
        n85 = flat-sequence {
          tunnel: w217 -> [w227]
          tunnel: w216 -> [w226]
          tunnel: [w223] -> w213
          tunnel: [w225] -> w211
          tunnel: [w224] -> w210
          tunnel: [w222] -> w209
          tunnel: w208 -> [w221]
          tunnel: [w229] -> w212
          tunnel: [w230] -> w214
          tunnel: [w231] -> w215
          tunnel: w211 -> [w231]
          tunnel: w210 -> [w230]
          tunnel: w209 -> [w229]
          frame #0 {
            n86 = call "Detect Finger.vi"("VISA Refnum in"=w227, "Cmd"="ï\u0001ÿÿÿÿ\u0001\u0000\u0004\u0002\u0001\u0000\b" ("write buffer"), "error in (no error)"=w226, "Buffer In"=w221) -> ("VISA Refnum out"=w225:refnum<visa-resource-name>, "Response"=w222:string, "Cmd Suceed?"=w223:bool, "error out"=w224:errorcluster)  [unwired: 6 in, 2 out]
          }
          frame #1 {
            n87 = disable-structure shown="Disabled" {
              frame Disabled {
                n88 = Wait (ms)(milliseconds to wait=u32 500) -> ()  [unwired: 1 out]
              }
              frame Enabled {
              }
            }
          }
        }
        n89 = Select(t=w220, s=w213, f=string[] []) -> (s? t:f=w219:string[])
      }
      frame "Get Image2" {
        # "EF01 FFFF FFFF 0100 0402 0200 09"
        n90 = flat-sequence {
          tunnel: w242 -> [w252]
          tunnel: w241 -> [w251]
          tunnel: [w248] -> w238
          tunnel: [w250] -> w236
          tunnel: [w249] -> w235
          tunnel: [w247] -> w234
          tunnel: w233 -> [w246]
          tunnel: [w254] -> w237
          tunnel: [w255] -> w239
          tunnel: [w256] -> w240
          tunnel: w236 -> [w256]
          tunnel: w235 -> [w255]
          tunnel: w234 -> [w254]
          frame #0 {
            n91 = call "Detect Finger.vi"("VISA Refnum in"=w252, "Cmd"="ï\u0001ÿÿÿÿ\u0001\u0000\u0004\u0002\u0002\u0000\t" ("write buffer"), "error in (no error)"=w251, "Buffer In"=w246) -> ("VISA Refnum out"=w250:refnum<visa-resource-name>, "Response"=w247:string, "Cmd Suceed?"=w248:bool, "error out"=w249:errorcluster)  [unwired: 6 in, 2 out]
          }
          frame #1 {
            n92 = disable-structure shown="Disabled" {
              frame Disabled {
                n93 = Wait (ms)(milliseconds to wait=u32 500) -> ()  [unwired: 1 out]
              }
              frame Enabled {
              }
            }
          }
        }
        n94 = Select(t=w245, s=w238, f=string[] []) -> (s? t:f=w244:string[])
      }
      frame "Merge Data" {
        n95 = call "Detect Finger.vi"("VISA Refnum in"=w265, "Cmd"="ï\u0001ÿÿÿÿ\u0001\u0000\u0003\u0005\u0000\t" ("write buffer"), "error in (no error)"=w264, "Buffer In"=w258) -> ("VISA Refnum out"=w263:refnum<visa-resource-name>, "Response"=w260:string, "Cmd Suceed?"=w261:bool, "error out"=w262:errorcluster)  [unwired: 6 in, 2 out]
        n96 = Select(t=w268, s=w261, f=string[] []) -> (s? t:f=w267:string[])
      }
      frame "Add Finger" {
        (unwired) "ï\u0001ÿÿÿÿ\u0001\u0000\u0006\u0006\u0002\u0000\u0000" ("write buffer")
        n97 = Unbundle By Name(w282) -> ("eRName"=w281:string, "eRClock"=w280:string)
        n98 = property on="Level" class="Enum (strict)"() -> ("RingText.Text"=w294:string)  [unwired: 2 in, 2 out]
        n99 = call <vilib>:"Trim Whitespace.vi"("string"=w280) -> ("trimmed string"=w277:string)  [unwired: 1 in]
        n100 = call <vilib>:"DB Tools Select Data.vi"("error in (no error)"=w303, "table"=w299, "connection reference"=w304) -> ("error out"=w300:errorcluster, "data"=w292:variant[][], "connection reference out"=w301:T5)  [unwired: 3 in]
        n101 = call <vilib>:"Trim Whitespace.vi"("string"=w281) -> ("trimmed string"=w278:string)  [unwired: 1 in]
        n102 = Variant To Data(type=string[][] [], Variant=w292) -> (data=w290:string[][])  [unwired: 1 in, 1 out]
        n103 = local read "Password"() -> (w274:string)
        n104 = Concatenate Strings(w278, "_" ("string"), w277) -> (w276:string)
        n105 = Index Array(array=w290, index (col)=0 ("disabled index (col)")) -> (element=w289:string[])  [unwired: 1 in]
        n106 = Decimal String To Number(string=w289) -> (number=w288:i32[])  [unwired: 2 in, 1 out]
        n107 = call <vilib>:"Trim Whitespace.vi"("string"=w274) -> ("trimmed string"=w273:string)  [unwired: 1 in]
        n108 = call <vilib>:"Trim Whitespace.vi"("string"=w276) -> ("trimmed string"=w275:string)  [unwired: 1 in]
        n109 = Get Date/Time In Seconds() -> (seconds since 1Jan1904=w295:timestamp)
        n110 = call "ID Generator.vi"("ID in"=w288) -> ("ID out"=w287:i32[])
        n111 = Index Array(array=w287) -> (element=w286:i32)  [unwired: 1 in]
        n112 = call <vilib>:"Trim Whitespace.vi"("string"="User Name") -> ("trimmed string"=w285:string)  [unwired: 1 in]
        n113 = To Unsigned Word Integer(number=w286) -> (unsigned 16bit integer=w271:u16)
        n114 = call <vilib>:"Trim Whitespace.vi"("string"="Clock No.") -> ("trimmed string"=w284:string)  [unwired: 1 in]
        n115 = call "Password.vi"("Password In"=w273) -> ("Password out"=w272:string)
        n116 = local read "Image Location"() -> (w270:path)
        n117 = disable-structure shown="Enabled" {
          disable-tunnel: w310 -> [w322 w325]
          disable-tunnel: w309 -> [w321 w324]
          disable-tunnel: [w320 w325] -> w308
          disable-tunnel: [w319 w324] -> w307
          disable-tunnel: [w318 _] -> w306
          disable-tunnel: w305 -> [w316 _]
          disable-tunnel: [w315 TRUE ("Cmd.")] -> w283
          disable-tunnel: w271 -> [w314 _]
          frame Disabled {
            n118 = call "Add Finger Cmd.vi"("ID NUMBER"=w314) -> ("Add Cmd"=w317:string)
            n119 = call "Detect Finger.vi"("VISA Refnum in"=w322, "Cmd"=w317, "error in (no error)"=w321, "Buffer In"=w316) -> ("VISA Refnum out"=w320:refnum<visa-resource-name>, "Response"=w318:string, "Cmd Suceed?"=w315:bool, "error out"=w319:errorcluster)  [unwired: 6 in, 2 out]
          }
          frame Enabled {
          }
        }
        n120 = local write "ID Number"(w271) -> ()
        n121 = Bundle By Name(cluster=T1 {"eRID"=0, "eRName"="", "eRClock"="", "eRDate"=timestamp(0 s since 1904-01-01), "eRLevel"="", "eRAdmin"="", "eRPassword"=""} ("Cluster"), "eRID"=w271, "eRName"=w285, "eRClock"=w284, "eRDate"=w295, "eRLevel"=w294, "eRAdmin"=w275, "eRPassword"=w272) -> (w269:T1)
        n122 = local write "Cmd."(w283) -> ()
        n123 = To Variant(anything=w269) -> (Variant=w293:variant)
        n124 = case shown="True" w283 {
          tunnel: w301 -> [_ w335]
          tunnel: w300 -> [_ w334]
          tunnel: w299 -> [_ w333]
          tunnel: w293 -> [_ w332]
          tunnel: [_ w330] -> _
          tunnel: w270 -> [_ w329]
          tunnel: w269 -> [_ w328]
          frame False {
          }
          frame True {
            w331 = "" ("Re-enter Password")
            n125 = call "Copy_eID_Image.vi"("eID_Details"=w328, "Image Location"=w329) -> ()  [unwired: 10 in]
            n126 = local write "Re-enter Password"(w331) -> ()
            n127 = local write "Password"(w331) -> ()
            n128 = call <vilib>:"DB Tools Insert Data.vi"("data"=w332, "error in (no error)"=w334, "table"=w333, "connection reference"=w335) -> ("error out"=w330:errorcluster)  [unwired: 6 in, 1 out]
            n129 = local write "Image Location"(path "" ("Image Location")) -> ()
            n130 = local write "Profile Image"(picture data[5B] ("Profile Image")) -> ()
          }
        }
        n131 = Select(t=w313, s=w283, f=string[] []) -> (s? t:f=w312:string[])
      }
      frame "Dummy" {
      }
      frame "Idle", Default {
        n132 = event shown="[1] \"Change Password\": Value Change" {
          selector: _ -> [_ _ _ _ _ _ _ _ _ _ _ _ _]
          dyn-events: _ -> [_ _ _ _ _ _ _ _ _ _ _ _ _]
          timeout: 100 -> [_ _ _ _ _ _ _ _ _ _ _ _ _]
          tunnel: w350 -> [w354 w397 w456 w468 w483 w486 w489 w497 _ _ w526 w539 w581]
          tunnel: [w354 w397 w456 w468 w483 w486 w489 w507 _ string[] ["Finger Presence1", "Get Image1", "Find Finger"] w529 w540 w581] -> w349
          tunnel: w348 -> [w353 w396 w455 w467 w482 w485 w488 w506 w514 w525 w531 w542 w580]
          tunnel: w347 -> [w352 w395 w454 w466 w481 w484 w487 w505 w513 w524 w530 w541 w579]
          tunnel: [w353 w396 w455 w467 w482 w485 w488 w506 w514 w525 w531 w542 w580] -> w346
          tunnel: [w352 w395 w454 w466 w481 w484 w487 w505 w513 w524 w530 w541 w579] -> w345
          tunnel: w343 -> [_ w379 _ w464 w479 _ _ _ _ _ _ _ w567]
          tunnel: w342 -> [_ w378 _ w463 w478 _ _ _ _ _ _ _ w566]
          tunnel: w341 -> [_ _ _ w462 _ _ _ _ _ _ _ _ _]
          tunnel: w340 -> [_ w360 _ _ _ _ _ _ _ _ _ w537 _]
          event Timeout {
            n133 = event-data() -> ()  [unwired: 1 in, 1 out]
          }
          event "Change Password": Value Change {
            n134 = event-data() -> ("CtlRef"=w373:refnum<vi>)  [unwired: 1 in]
            n135 = local read "ID Number"() -> (w358:i16)
            n136 = Format Into String(format string="SELECT *  FROM [dbo].[User_Management] Where [eRID] = '%d'" ("SQL query"), w358) -> (resulting string=w389:string)  [unwired: 2 in, 1 out]
            n137 = call-poly <vilib>:"DB Tools Execute Query.vi"("error in (no error)"=w378, "SQL query"=w389, "connection reference"=w379) -> ("error out"=w388:errorcluster, "recordset reference"=w391:T8)  [unwired: 5 in]
            n138 = call-poly <vilib>:"DB Tools Fetch Recordset Data.vi"("error in (no error)"=w388, "recordset reference"=w391) -> ("error out"=w393:errorcluster, "recordset data"=w381:variant[][], "recordset reference out"=w392:T8)  [unwired: 3 in]
            n139 = local read "User Name"() -> (w357:string)
            n140 = local read "Clock No."() -> (w356:string)
            n141 = Index Array(array=w381, index (row)=0 ("disabled index (col)")) -> (element=w387:variant[])  [unwired: 1 in]
            n142 = call-poly <vilib>:"DB Tools Free Object.vi"("error in (no error)"=w393, "recordset reference"=w392) -> ("error out"=w375:errorcluster, "connection reference"=w363:T5)  [unwired: 8 in]
            n143 = local read "Password"() -> (w369:string)
            n144 = local read "Re-enter Password"() -> (w368:string)
            n145 = Variant To Data(type=string[] [], Variant=w387) -> (data=w385:string[])  [unwired: 1 in, 1 out]
            n146 = call <vilib>:"Clear Errors.vi"("error in (no error)"=w375) -> ("error out"=w370:errorcluster)  [unwired: 5 in, 1 out]
            n147 = local read "Auth. Password"() -> (w377:string)
            n148 = Index Array(array=w385, index=6) -> (element=w383:string)
            n149 = call <vilib>:"Trim Whitespace.vi"("string"=w369) -> ("trimmed string"=w362:string)  [unwired: 1 in]
            n150 = call <vilib>:"Trim Whitespace.vi"("string"=w368) -> ("trimmed string"=w367:string)  [unwired: 1 in]
            n151 = call <vilib>:"Trim Whitespace.vi"("string"=w383) -> ("trimmed string"=w382:string)  [unwired: 1 in]
            n152 = call "Password.vi"("Password In"=w382) -> ("Password out"=w380:string)
            n153 = Equal?(x=w362, y=w367) -> (x = y?=w366:bool)
            n154 = Empty String/Path?(string/path=w367) -> (empty?=w365:bool)
            n155 = Format Into String(format string="%d_%s_%s Password Changed", w358, w357, w356) -> (resulting string=w355:string)  [unwired: 2 in, 1 out]
            n156 = Equal?(x=w377, y=w380) -> (x = y?=w376:bool)
            n157 = Compound Arithmetic op=AND(w366, invert w365) -> (w364:bool)
            n158 = case shown="True" w376 {
              tunnel: [w399 w405] -> w371
              tunnel: w370 -> [w399 w408]
              tunnel: w364 -> [_ w411]
              tunnel: w363 -> [_ w410]
              tunnel: w362 -> [_ w409]
              tunnel: "UPDATE [dbo].[User_Management]\n   SET [eRPassword] = '%s'\n WHERE [eRID] = '%d'" ("SQL query") -> [_ w407]
              tunnel: w358 -> [_ w406]
              tunnel: w360 -> [_ w404]
              tunnel: w355 -> [_ w403]
              frame False {
                n159 = property on="Hide" class="Bool"("Visible"=TRUE) -> (error out=w398:errorcluster)  [unwired: 2 in, 1 out]
                n160 = flat-sequence {
                  tunnel: "Password Authentication Fail." ("resulting string") -> [w402]
                  tunnel: w398 -> [_]
                  frame #0 {
                    n161 = call <userlib>:"Warning .vi"("Warning in"=w402) -> ()  [unwired: 15 in]
                  }
                }
              }
              frame True {
                n162 = case shown="True" w411 {
                  tunnel: w410 -> [_ w443]
                  tunnel: w409 -> [_ w444]
                  tunnel: w408 -> [_ w434]
                  tunnel: w407 -> [_ w442]
                  tunnel: w406 -> [_ w440]
                  tunnel: [_ w422] -> w405
                  tunnel: w404 -> [_ w421]
                  tunnel: w403 -> [_ w416]
                  frame False {
                    n163 = property on="Hide" class="Bool"("Visible"=TRUE) -> (error out=w412:errorcluster)  [unwired: 2 in, 1 out]
                    n164 = flat-sequence {
                      tunnel: "New Password Mismatch or Invalid." ("resulting string") -> [w415]
                      tunnel: w412 -> [_]
                      frame #0 {
                        n165 = call <userlib>:"Warning .vi"("Warning in"=w415) -> ()  [unwired: 15 in]
                      }
                    }
                  }
                  frame True {
                    n166 = call "Password.vi"("Password In"=w444) -> ("Password out"=w441:string)
                    n167 = property on="Hide" class="Bool"(error in=w434, "Visible"=TRUE) -> (error out=w433:errorcluster)  [unwired: 1 in, 1 out]
                    n168 = Format Into String(format string=w442, w441, w440) -> (resulting string=w439:string)  [unwired: 2 in, 1 out]
                    n169 = call-poly <vilib>:"DB Tools Execute Query.vi"("error in (no error)"=w433, "SQL query"=w439, "connection reference"=w443) -> ("error out"=w437:errorcluster, "recordset reference"=w438:T8)  [unwired: 5 in]
                    n170 = call-poly <vilib>:"DB Tools Free Object.vi"("error in (no error)"=w437, "recordset reference"=w438) -> ("error out"=w436:errorcluster, "connection reference"=w424:T5)  [unwired: 8 in]
                    n171 = call <vilib>:"Clear Errors.vi"("error in (no error)"=w436) -> ("error out"=w423:errorcluster)  [unwired: 5 in, 1 out]
                    n172 = flat-sequence {
                      tunnel: w436 -> [_]
                      tunnel: "Password Changed." ("resulting string") -> [w445]
                      frame #0 {
                        n173 = call <userlib>:"Warning .vi"("Warning in"=w445) -> ()  [unwired: 15 in]
                      }
                    }
                    n174 = Unbundle By Name(w421) -> ("eRID"=w420:u16, "eRName"=w419:string, "eRClock"=w418:string, "eRLevel"=w417:string)  [unwired: 1 out]
                    n175 = Get Date/Time In Seconds() -> (seconds since 1Jan1904=w429:timestamp)
                    n176 = Bundle By Name(cluster=T7 {"eRID"=0, "eRName"="", "eRClock"="", "eRDate"=timestamp(0 s since 1904-01-01), "eRLevel"="", "eRAdmin"="", "eRPassword"="", "eRPurpose"=""} ("Cluster"), "eRID"=w420, "eRName"=w419, "eRClock"=w418, "eRDate"=w429, "eRLevel"=w417, "eRAdmin"="", "eRPassword"="Password", "eRPurpose"=w416) -> (w430:T7)
                    n177 = To Variant(anything=w430) -> (Variant=w431:variant)
                    n178 = call <vilib>:"DB Tools Insert Data.vi"("data"=w431, "error in (no error)"=w423, "table"="UserLogin", "connection reference"=w424) -> ("error out"=w422:errorcluster)  [unwired: 6 in, 1 out]
                  }
                }
              }
            }
            n179 = property class="Bool (strict)"(reference=w373, error in=w371, "Value"=FALSE) -> ()  [unwired: 2 out]
            n180 = property on="Hide" class="Bool"(error in=w371, "Visible"=FALSE) -> ()  [unwired: 1 in, 2 out]
          }
          event "Image Location": Value Change {
            n181 = event-data() -> ("NewVal"=w450:path)  [unwired: 1 in]
            n182 = call "Open_Image.vi"("NewVal"=w450) -> ("image data"=w452:T9)  [unwired: 10 in]
            n183 = property on="Profile Image" class="Pict"() -> ("Draw Area Size"=w449:T10)  [unwired: 2 in, 2 out]
            n184 = Unbundle By Name(w452) -> ("Rectangle"=w453:T11)
            n185 = Unbundle By Name(w449) -> ("Width"=w447:u32)
            n186 = call <vilib>:"Draw Flattened Pixmap.vi"("image data"=w452) -> ("new picture"=→"Profile Image":picture)  [unwired: 8 in]
            n187 = Unbundle By Name(w453) -> ("right"=w448:i16)
            n188 = Divide(x=w447, y=w448) -> (x/y=w446:dbl)
            n189 = property on="Profile Image" class="Pict"("ZoomFactor"=w446) -> ()  [unwired: 2 in, 2 out]
          }
          event "View All": Value Change {
            n190 = event-data() -> ("CtlRef"=w461:refnum<vi>)  [unwired: 1 in]
            n191 = call <vilib>:"DB Tools Select Data.vi"("condition"="Order By eRDate", "error in (no error)"=w463, "table"=w462, "connection reference"=w464) -> ("error out"=w457:errorcluster, "data"=w465:variant[][])  [unwired: 2 in, 1 out]
            n192 = flat-sequence {
              tunnel: w465 -> [w471]
              tunnel: [errorcluster {"status"=FALSE, "code"=0, "source"=""} ("error in (no error)")] -> w460
              tunnel: w457 -> [_]
              frame #0 {
                n193 = call "1775E_User List.vi"("Log?"=TRUE, "data"=w471) -> ()  [unwired: 10 in]
              }
            }
            n194 = property class="Bool (strict)"(reference=w461, error in=w460, "Value"=FALSE) -> ()  [unwired: 2 out]
          }
          event "View Log": Value Change {
            n195 = event-data() -> ("CtlRef"=w477:refnum<vi>)  [unwired: 1 in]
            n196 = call <vilib>:"DB Tools Select Data.vi"("condition"="Order By eRDate Desc", "error in (no error)"=w478, "table"="UserLogin", "connection reference"=w479) -> ("error out"=w472:errorcluster, "data"=w480:variant[][])  [unwired: 2 in, 1 out]
            n197 = call "1775E_Login List.vi"("error in (no error)"=w472, "data"=w480) -> ("error out"=w476:errorcluster)  [unwired: 9 in]
            n198 = property class="Bool (strict)"(reference=w477, error in=w476, "Value"=FALSE) -> ()  [unwired: 2 out]
          }
          event "Super User": Value Change {
            n199 = event-data() -> ()  [unwired: 1 in, 1 out]
          }
          event "Stop": Value Change {
            n200 = event-data() -> ()  [unwired: 1 in, 1 out]
          }
          event "Enroll": Value Change {
            n201 = event-data() -> ()  [unwired: 1 in, 1 out]
            n202 = local read "Clock No."() -> (w503:string)
            n203 = local read "User Name"() -> (w504:string)
            n204 = local read "Password"() -> (w491:string)
            n205 = local read "Re-enter Password"() -> (w495:string)
            n206 = call <vilib>:"Trim Whitespace.vi"("string"=w503) -> ("trimmed string"=w502:string)  [unwired: 1 in]
            n207 = call <vilib>:"Trim Whitespace.vi"("string"=w504) -> ("trimmed string"=w501:string)  [unwired: 1 in]
            n208 = call <vilib>:"Trim Whitespace.vi"("string"=w491) -> ("trimmed string"=w494:string)  [unwired: 1 in]
            n209 = call <vilib>:"Trim Whitespace.vi"("string"=w495) -> ("trimmed string"=w493:string)  [unwired: 1 in]
            n210 = Empty String/Path?(string/path=w491) -> (empty?=w490:bool)
            n211 = Not Equal?(x=w494, y=w493) -> (x != y?=w492:bool)
            n212 = Empty String/Path?(string/path=w502) -> (empty?=w500:bool)
            n213 = Empty String/Path?(string/path=w501) -> (empty?=w499:bool)
            n214 = Compound Arithmetic op=OR(w500, w499, w492, w490) -> (w498:bool)
            n215 = case shown="False" w498 {
              selector: w498 -> [w508 _]
              tunnel: [string[] ["Add Finger"] w512] -> w507
              tunnel: w497 -> [_ w512]
              tunnel: [w508 FALSE] -> w496
              frame False {
              }
              frame True {
                n216 = call <userlib>:"Warning .vi"("Warning in"="Empty User Name or Clock No. or Invalid Password.!") -> ()  [unwired: 15 in]
              }
            }
            n217 = local write "Enroll"(w496) -> ()
          }
          event "Password", "Re-enter Password": Value Change {
            n218 = event-data() -> ("CtlRef"=w516:refnum<vi>, "NewVal"=w520:string)  [unwired: 1 in, 1 out]
            n219 = call <vilib>:"Trim Whitespace.vi"("string"=w520) -> ("trimmed string"=w519:string)  [unwired: 1 in]
            n220 = String Subset(string=w519, offset (0)=0, length (rest)=8 ("length (rest)")) -> (substring=w515:string)
            n221 = property class="Str"(reference=w516, "Value"=w515) -> ()  [unwired: 1 in, 2 out]
          }
          event "Search": Value Change {
            w521 = "" ("User Name")
            (unwired) "Search"
            n222 = event-data() -> ()  [unwired: 1 in, 1 out]
            n223 = local write "User Name"(w521) -> ()
            n224 = local write "Clock No."(w521) -> ()
            n225 = local write "ID Number"(i16 -1 ("ID")) -> ()
          }
          event "Delete All": Value Change {
            n226 = event-data() -> ()  [unwired: 1 in, 1 out]
            n227 = call <userlib>:"Warning With option(W).vi"("Warning in"="Are you sure you want to Delete all Users?") -> ("Cancel ?"=w527:bool)  [unwired: 13 in, 1 out]
            n228 = case shown="False" w527 {
              tunnel: [string[] ["Delete All"] w533] -> w529
              tunnel: w526 -> [_ w533]
              frame False {
              }
              frame True {
              }
            }
          }
          event "Delete": Value Change {
            (unwired) "Search"
            n229 = event-data() -> ()  [unwired: 1 in, 1 out]
            n230 = local read "ID Number"() -> (w535:i16)
            n231 = Unbundle By Name(w537) -> ("eRID"=w536:u16)
            n232 = Equal?(x=w535, y=w536) -> (x = y?=w534:bool)
            n233 = case shown="False" w534 {
              tunnel: [w547 w553] -> w540
              tunnel: w539 -> [w544 w553]
              tunnel: [w543 FALSE] -> w538
              frame False {
                n234 = call <userlib>:"Warning With option(W).vi"("Warning in"="Are you sure you want to Delete this User ID?") -> ("Cancel ?"=w545:bool)  [unwired: 13 in, 1 out]
                n235 = case shown="False" w545 {
                  selector: w545 -> [w548 _]
                  tunnel: [string[] ["Delete ID"] w550] -> w547
                  tunnel: w544 -> [_ w550]
                  tunnel: [w548 _] -> w543
                  frame False {
                  }
                  frame True {
                  }
                }
              }
              frame True {
                n236 = call <userlib>:"Warning .vi"("Warning in"="This ID is used for Login. Can't able to Delete.") -> ()  [unwired: 15 in]
              }
            }
            n237 = local write "Delete"(w538) -> ()
          }
          event "ID Number": Value Change {
            n238 = event-data() -> ("NewVal"=w568:i16)  [unwired: 1 in]
            n239 = Format Into String(format string="SELECT [eRClock],[eRLevel],[eRName] FROM [dbo].[User_Management] where [eRID] = '%d' order by [eRClock] asc" ("Response"), w568) -> (resulting string=w574:string)  [unwired: 2 in, 1 out]
            n240 = call-poly <vilib>:"DB Tools Execute Query.vi"("error in (no error)"=w566, "SQL query"=w574, "connection reference"=w567) -> ("error out"=w573:errorcluster, "recordset reference"=w576:T8)  [unwired: 5 in]
            n241 = call-poly <vilib>:"DB Tools Fetch Recordset Data.vi"("error in (no error)"=w573, "recordset reference"=w576) -> ("error out"=w578:errorcluster, "recordset data"=w570:variant[][], "recordset reference out"=w577:T8)  [unwired: 3 in]
            n242 = Index Array(array=w570, index (row)=0 ("disabled index (col)")) -> (element=w572:variant[])  [unwired: 1 in]
            n243 = call-poly <vilib>:"DB Tools Free Object.vi"("error in (no error)"=w578, "recordset reference"=w577) -> ()  [unwired: 8 in, 2 out]
            n244 = Variant To Data(type=string[] [], Variant=w572) -> (data=w559:string[])  [unwired: 1 in, 1 out]
            n245 = Index Array(array=w559) -> (element #1=w561:string, element #2=w564:string, element #3=w560:string)  [unwired: 3 in]
            n246 = Empty Array?(array=w559) -> (empty?=w556:bool)
            n247 = call <vilib>:"Trim Whitespace.vi"("string"=w564) -> ("trimmed string"=w565:string)  [unwired: 1 in]
            n248 = local write "User Name"(w560) -> ()
            n249 = local write "Clock No."(w561) -> ()
            n250 = Not(x=w556) -> (.not. x?=w558:bool)
            n251 = property on="Level" class="Enum (strict)"() -> ("Strings []"=w563:string[])  [unwired: 2 in, 2 out]
            n252 = Select(t="Password" ("element"), s=w556, f="New Password" ("element")) -> (s? t:f=w554:string)
            n253 = property on="Enroll" class="Bool (strict)"("Visible"=w556) -> ()  [unwired: 2 in, 2 out]
            n254 = property on="Change Password" class="Bool (strict)"("Visible"=w558) -> ()  [unwired: 2 in, 2 out]
            n255 = Search 1D Array(1D array=w563, element=w565) -> (index of element=w562:i32)  [unwired: 1 in]
            n256 = property on="Auth. Password" class="Str"("Visible"=w558) -> ()  [unwired: 2 in, 2 out]
            n257 = property on="Password" class="Str"("Caption.Text"=w554) -> ()  [unwired: 2 in, 2 out]
            n258 = local write "Level"(w562) -> ()
          }
        }
      }
      frame "Init" {
        n259 = stacked-sequence {
          tunnel: [_ w604] -> w589
          tunnel: w588 -> [_ w603]
          tunnel: [_ w602] -> w587
          tunnel: w586 -> [_ w601]
          tunnel: w585 -> [_ w599]
          tunnel: [_ w598] -> w584
          tunnel: [_ w594] -> _
          tunnel: [w591 _] -> w582
          frame #0 {
            n260 = invoke class="VI" method="Default Vals.Reinit All"() -> (error out=w591:errorcluster)  [unwired: 3 in, 2 out]
          }
          frame #1 {
            w593 = "" ("User Name")
            n261 = property on="Level" class="Enum (strict)"("Disabled Items []"=i32[] [4]) -> ()  [unwired: 2 in, 2 out]
            n262 = call "Detect Finger.vi"("VISA Refnum in"=w603, "Cmd"="ï\u0001ÿÿÿÿ\u0001\u0000\u0003\u0016\u0000\u001a", "error in (no error)"=w599, "Buffer In"=w601) -> ("VISA Refnum out"=w602:refnum<visa-resource-name>, "Cmd Suceed?"=w594:bool, "Buffer Out"=w600:string, "error out"=w598:errorcluster)  [unwired: 6 in, 2 out]
            n263 = property on="ID Number" class="DigNum (strict)"("Val(Sgnl)"=i16 -1 ("ID")) -> ()  [unwired: 2 in, 2 out]
            n264 = call "Get Device Info.vi"("Read Data"=w600) -> ("Device Info"=w604:string)
            "Device Info" <- w604
            n265 = local write "Re-enter Password"(w593) -> ()
            n266 = local write "Password"(w593) -> ()
            n267 = local write "User Name"(w593) -> ()
            n268 = local write "Clock No."(w593) -> ()
            "Cmd." <- FALSE ("Cmd.")
          }
        }
        n269 = property on="Hide" class="Bool"(error in=w582, "Visible"=FALSE) -> ()  [unwired: 1 in, 2 out]
      }
    }
    "Response" <- w57
    n270 = Compound Arithmetic op=OR(w60, "Stop") -> (w62:bool)
    "Numeric" <- w52
  }
  n271 = VISA Close(VISA resource name=w19, error in (no error)=w18) -> (error out=w17:errorcluster)
  n272 = call <vilib>:"Clear Errors.vi"("error in (no error)"=w17) -> ()  [unwired: 5 in, 2 out]
